vi "m1m3_putSample_PIDData.vi"(8 "error in (no error)":errorcluster, 11 "PIDData_Ctl":T1={"Timestamp"=0.0, "Setpoint[6]"=[0.0, 0.0, 0.0, 0.0, 0.0, 0.0], "Measurement[6]"=[0.0, 0.0, 0.0, 0.0, 0.0, 0.0], "Error[6]"=[0.0, 0.0, 0.0, 0.0, 0.0, 0.0], "ErrorT1[6]"=[0.0, 0.0, 0.0, 0.0, 0.0, 0.0], "ErrorT2[6]"=[0.0, 0.0, 0.0, 0.0, 0.0, 0.0], "Control[6]"=[0.0, 0.0, 0.0, 0.0, 0.0, 0.0], "ControlT1[6]"=[0.0, 0.0, 0.0, 0.0, 0.0, 0.0], "ControlT2[6]"=[0.0, 0.0, 0.0, 0.0, 0.0, 0.0]}) -> (0 "error out":errorcluster, 2 "function return":i32, 3 "PIDData_Ctl out":T1)   [LabVIEW 2016, in "SALLV_m1m3.lvlib"]
doc: "int m1m3_shm_putSample_PIDDataLV(m1m3_PIDDataLV *PIDData_Ctl );"
uses:
  SALLV_m1m3.lvlib
  DataTypes/PIDData.ctl
  SALLV_m1m3.so
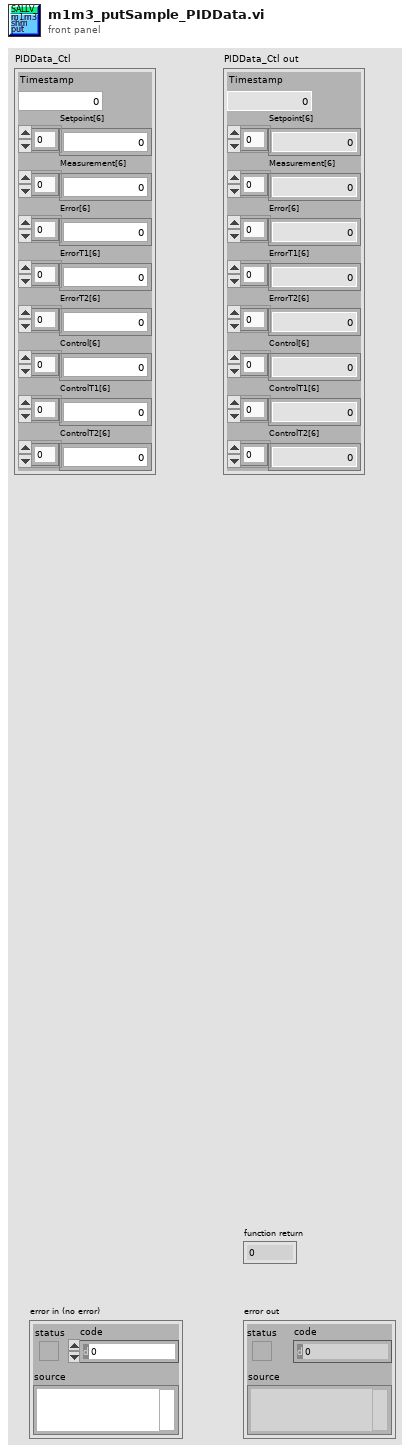
[diagram p1: front panel]
types:
  T1 = typedef "SALLV_m1m3.lvlib/PIDData.ctl" = cluster{"Timestamp":dbl, "Setpoint[6]":dbl[], "Measurement[6]":dbl[], "Error[6]":dbl[], "ErrorT1[6]":dbl[], "ErrorT2[6]":dbl[], "Control[6]":dbl[], "ControlT1[6]":dbl[], "ControlT2[6]":dbl[]}
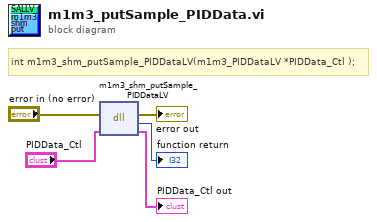
[diagram p0: block diagram]
diagram:
  # "int m1m3_shm_putSample_PIDDataLV(m1m3_PIDDataLV *PIDData_Ctl );"
  n1 = dll-call lib="opt/CODE/SALLV_m1m3/SALLV_m1m3.*" fn="m1m3_shm_putSample_PIDDataLV"(error in="error in (no error)", "PIDData_Ctl"="PIDData_Ctl") -> (error out=→"error out":errorcluster, →"function return":i32, "PIDData_Ctl"=→"PIDData_Ctl out":T1)  [unwired: 2 in, 1 out]
